vi "GVSView Close.vi"   [LabVIEW 2013]
panel:
  # "Close View."
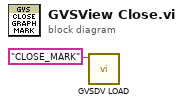
[diagram p0: block diagram]
diagram:
  n1 = call "GVSDV LOAD.vi"("sAction"="CLOSE_MARK") -> ()  [unwired: 7 in, 4 out]
